vi "Load Config.vi"(8 "error in (no error)":errorcluster, 11 "CurrentOutChannel in":refnum<class "CurrentOutChannel.lvclass">) -> (0 "error out":errorcluster, 3 "CurrentOutChannel out":refnum<class "CurrentOutChannel.lvclass">)   [LabVIEW 2020, in "VolatusDAQConfig.lvlib" / "CurrentOutChannel.lvclass"]
uses:
  CurrentOutChannel.lvclass
  CurrentOutChannel.lvclass/CurrentOutChannel.ctl
  VolatusConfig/VolatusConfigElement/VolatusConfigElement.lvclass
  lv-cdm/CDM-Config/Config Element/Config Element.lvclass
  C:/dev/lv20CE/relink/lv-volatus/VolatusDAQConfig/DAQmxChannel/DAQmxChannel.lvclass
  C:/dev/lv20CE/relink/lv-volatus/VolatusConfig/Channel/Channel.lvclass
  C:/dev/lv20CE/relink/lv-volatus/VolatusConfig/VolatusConfigElement/VolatusConfigElement.lvclass
  C:/dev/lv20CE/relink/lv-volatus/VolatusDAQConfig/CurrentOutChannel/CurrentOutChannel.lvclass
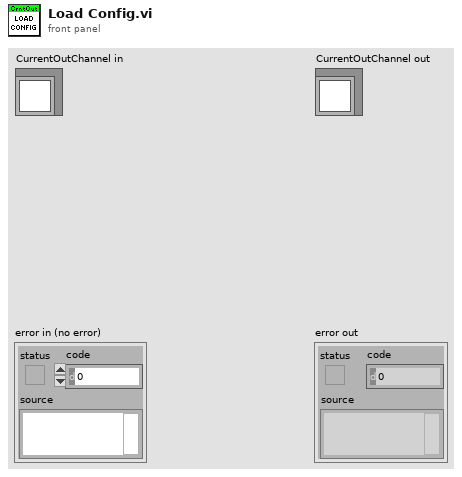
[diagram p1: front panel]
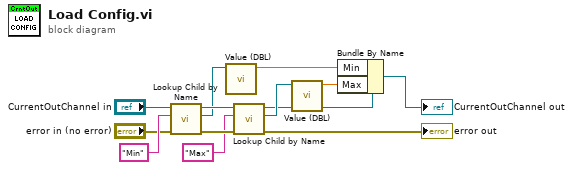
[diagram p0: block diagram]
diagram:
  n1 = call "Lookup Child by Name.vi"("error in (no error)"="error in (no error)", "Child Name"="Min", "VolatusConfigElement in"="CurrentOutChannel in") -> ("error out"=w13:errorcluster, "Child"=w10:refnum<class "Config Element.lvclass">, "VolatusConfigElement out"=w12:refnum<class "CurrentOutChannel.lvclass">)  [unwired: 5 in, 1 out]
  n2 = call "Value (DBL).vi"("Config Element in"=w10) -> ("DBL Value"=w4:dbl)  [unwired: 9 in, 1 out]
  n3 = call "Lookup Child by Name.vi"("error in (no error)"=w13, "Child Name"="Max", "VolatusConfigElement in"=w12) -> ("error out"=→"error out":errorcluster, "Child"=w9:refnum<class "Config Element.lvclass">, "VolatusConfigElement out"=w5:refnum<class "CurrentOutChannel.lvclass">)  [unwired: 5 in, 1 out]
  n4 = call "Value (DBL).vi"("Config Element in"=w9) -> ("DBL Value"=w3:dbl)  [unwired: 9 in, 1 out]
  n5 = Bundle By Name(cluster=w5, "Min"=w4, "Max"=w3) -> (→"CurrentOutChannel out":refnum<class "CurrentOutChannel.lvclass">)
